vi "Set Barcode Required.vi"(8 "ErrorIn":errorcluster, 10 "Command":string, 11 "VISAIn":refnum<visa-resource-name>) -> (0 "ErrorOut":errorcluster, 3 "VISAOut":refnum<visa-resource-name>)   [LabVIEW 2017, in "I28Drivers.lvlib"]
uses:
  I28Drivers.lvlib
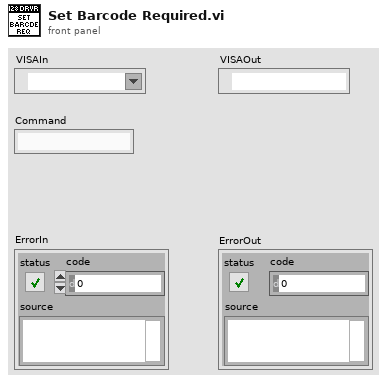
[diagram p1: front panel]
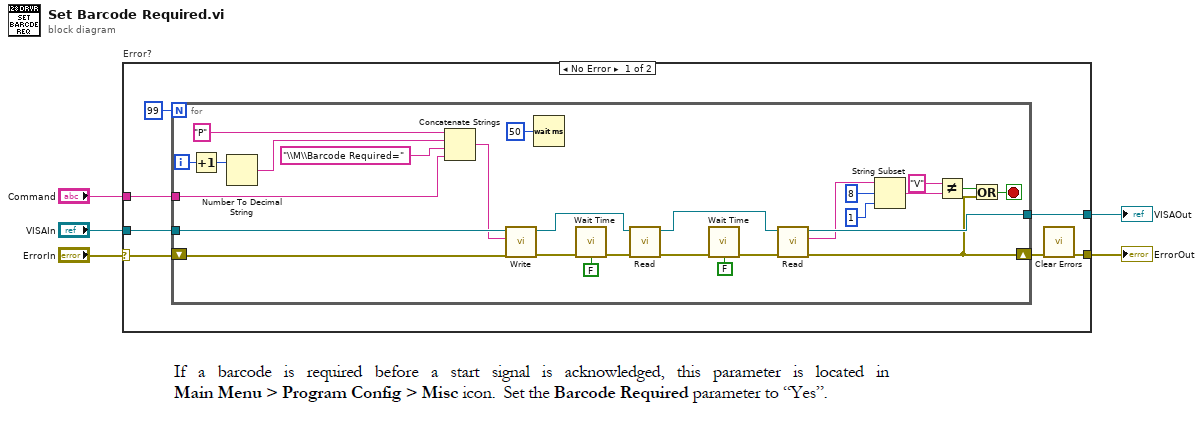
[diagram p0: block diagram]
diagram:
  n1 = case "Error?" shown="No Error" "ErrorIn" {
    selector: "ErrorIn" -> [w10 w41]
    tunnel: "VISAIn" -> [w11 w40]
    tunnel: "Command" -> [w12 _]
    tunnel: [w6 w41] -> w2
    tunnel: [w8 w40] -> w1
    frame No Error {
      n2 = for {
        N: 99 -> [_]
        tunnel: w12 -> [w34]
        tunnel: w11 -> [w33]
        tunnel: [w29] -> w8
        shift-right: [w13] -> w7
        shift-left: w10 -> [w32]
        i -> [w39]
        stop <- w14 stop-if-true
        n3 = Increment(x=w39) -> (x+1=w38:i32)
        n4 = Number To Decimal String(number=w38) -> (decimal integer string=w36:string)  [unwired: 1 in]
        n5 = Concatenate Strings("P", w36, "\\M\\Barcode Required=" ("string"), w34) -> (w31:string)
        n6 = call "Write.vi"("ErrorIn"=w32, "Command"=w31, "VISAIn"=w33) -> ("ErrorOut"=w21:errorcluster, "VISAOut"=w22:refnum<visa-resource-name>)  [unwired: 7 in]
        n7 = Wait (ms)(milliseconds to wait=u32 50) -> ()  [unwired: 1 out]
        n8 = call "Wait Time.vi"("error in"=w21, "Set Time"=FALSE) -> ("error out"=w20:errorcluster)  [unwired: 13 in]
        n9 = call "Read.vi"("ErrorIn"=w20, "VISAIn"=w22) -> ("ErrorOut"=w17:errorcluster, "VISAOut"=w18:refnum<visa-resource-name>)  [unwired: 7 in, 1 out]
        n10 = call "Wait Time.vi"("error in"=w17, "Set Time"=FALSE) -> ("error out"=w16:errorcluster)  [unwired: 13 in]
        n11 = call "Read.vi"("ErrorIn"=w16, "VISAIn"=w18) -> ("ErrorOut"=w13:errorcluster, "Data"=w28:string, "VISAOut"=w29:refnum<visa-resource-name>)  [unwired: 7 in]
        n12 = String Subset(string=w28, offset (0)=8, length (rest)=1 ("length (rest)")) -> (substring=w25:string)
        n13 = Not Equal?(x="V", y=w25) -> (x != y?=w23:bool)
        n14 = Or(x=w23, y=w13) -> (x .or. y?=w14:bool)
      }
      n15 = call <vilib>:"Clear Errors.vi"("error in (no error)"=w7) -> ("error out"=w6:errorcluster)  [unwired: 5 in, 1 out]
    }
    frame Error {
    }
  }
  "ErrorOut" <- w2
  "VISAOut" <- w1
